vi "Average samples.vi"(6 "wait for reply (T)":bool=TRUE, 8 "error in":errorcluster, 9 "N samples":i32, 10 "Parameter":u16, 11 "Module ID":i32=-1) -> (0 "error out":errorcluster, 1 "timed out?":bool, 3 "Measurement":dbl)   [LabVIEW 2020, in "Lock-in amplifier.lvlib"]
doc: "Request to acquire multiple samples from the device. Returns the simple average of the samples.\n_____\nCreated using DQMH Event Scripter 6.1.0.128."
uses:
  Lock-in amplifier.lvlib
  Average samples Argument--cluster.ctl
  Average samples (Reply Payload)--cluster.ctl
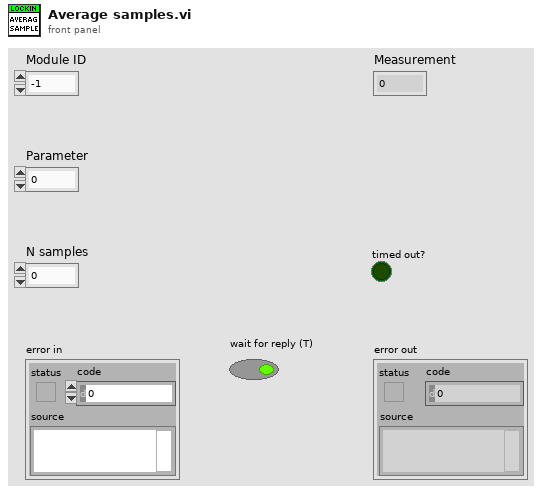
[diagram p1: front panel]
types:
  T1 = typedef "Lock-in amplifier.lvlib/Average samples Argument--cluster.ctl" = cluster{"Module ID":i32, "Parameter":u16, "N samples":i32, "Wait Notifier":refnum<notifier>, "wait for reply":bool}
  T2 = typedef "Lock-in amplifier.lvlib/Request Events--cluster.ctl" = cluster{"Stop Module":refnum<user-event>, "Show Panel":refnum<user-event>, "Hide Panel":refnum<user-event>, "Show Diagram":refnum<user-event>, "Get Module Execution Status":refnum<user-event>, "Draw Panel into Subpanel":refnum<user-event>, "Remove Panel from Subpanel":refnum<user-event>, "Connect":refnum<user-event>, "Read datapoint":refnum<user-event>, "Average samples":refnum<user-event>}
  T3 = typedef "Lock-in amplifier.lvlib/Average samples (Reply Payload)--cluster.ctl" = cluster{"Measurement":dbl, "error":errorcluster}
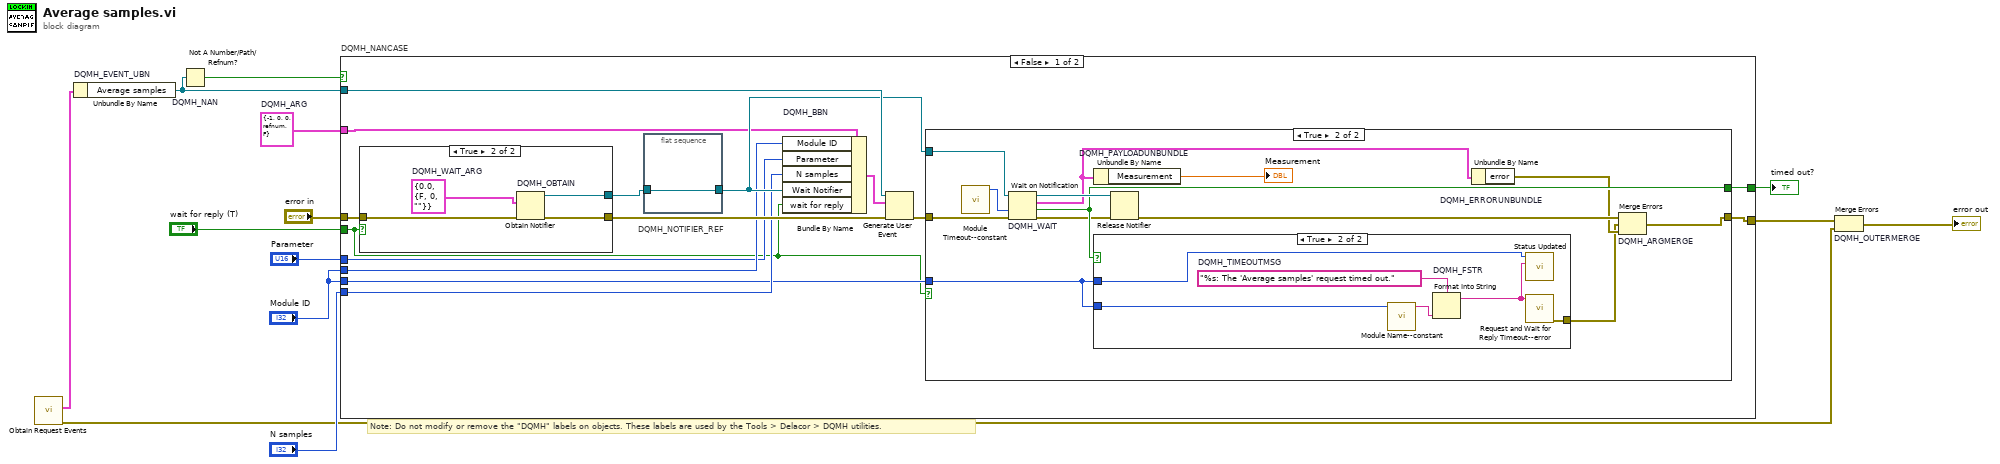
[diagram p0: block diagram]
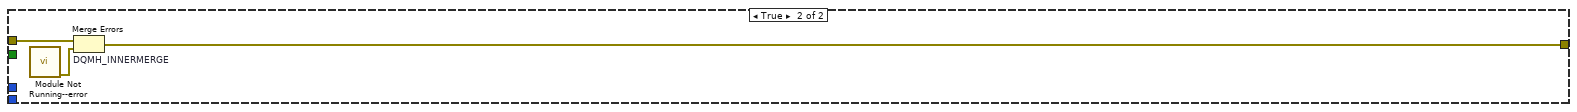
[diagram p5: hidden frame]
diagram:
  w7 = T1 {"Module ID"=-1, "Parameter"=0, "N samples"=0, "Wait Notifier"=refnum, "wait for reply"=FALSE}  # DQMH_ARG
  # "Note: Do not modify or remove the \"DQMH\" labels on objects. These labels are used by the Tools > Delacor > DQMH utilities."
  n1 = call "Obtain Request Events.vi"() -> ("error out"=w2:errorcluster, "Lock-in amplifier Request Events"=w1:T2)  [unwired: 10 in]
  n2 = Unbundle By Name "DQMH_EVENT_UBN"(w1) -> ("Average samples"=w11:refnum<user-event>)
  n3 = Not A Number/Path/Refnum? "DQMH_NAN"(number/path/refnum=w11) -> (NaN/Path/Refnum?=w10:bool)
  n4 = case "DQMH_NANCASE" shown="False" w10 {
    tunnel: "error in" -> [w28 w57]
    tunnel: w11 -> [w26 _]
    tunnel: [w23 w56] -> w8
    tunnel: [w24 _] -> w9
    tunnel: w7 -> [w19 _]
    tunnel: "Module ID" -> [w18 _]
    tunnel: "Parameter" -> [w17 _]
    tunnel: "N samples" -> [w16 _]
    tunnel: "Module ID" -> [w15 _]
    tunnel: "wait for reply (T)" -> [w14 _]
    frame False {
      n5 = case shown="True" w14 {
        tunnel: w28 -> [w50 w54]
        tunnel: [w50 w53] -> w25
        tunnel: [_ w51] -> w21
        frame False {
        }
        frame True {
          w52 = T3 {"Measurement"=0.0, "error"={"status"=FALSE, "code"=0, "source"=""}}  # DQMH_WAIT_ARG
          n6 = Obtain Notifier "DQMH_OBTAIN"(notification data type=w52, error in (no error)=w54) -> (notifier out=w51:refnum<notifier>, error out=w53:errorcluster)  [unwired: 2 in, 1 out]
        }
      }
      n7 = flat-sequence "DQMH_NOTIFIER_REF" {
        tunnel: w21 -> [w29]
        tunnel: [w29] -> w20
        frame #0 {
        }
      }
      n8 = Bundle By Name "DQMH_BBN"(cluster=w19, "Module ID"=w18, "Parameter"=w17, "N samples"=w16, "Wait Notifier"=w20, "wait for reply"=w14) -> (w22:T1)
      n9 = Generate User Event(user event=w26, event data cluster=w22, error in=w25) -> (error out=w27:errorcluster)  [unwired: 1 in, 1 out]
      n10 = case shown="True" w14 {
        tunnel: w27 -> [w30 w43]
        tunnel: w20 -> [_ w42]
        tunnel: [_ w40] -> w24
        tunnel: [w30 w39] -> w23
        tunnel: w15 -> [_ w31]
        frame False {
        }
        frame True {
          n11 = call "Module Timeout--constant.vi"() -> ("Module Timeout"=w33:i32)  [unwired: 11 in]
          n12 = Wait on Notification "DQMH_WAIT"(notifier=w42, timeout in ms (-1)=w33, error in (no error)=w43) -> (notifier out=w41:refnum<notifier>, notification=w34:T3, timed out?=w40:bool, error out=w38:errorcluster)  [unwired: 1 in]
          n13 = Unbundle By Name "DQMH_PAYLOADUNBUNDLE"(w34) -> ("Measurement"=→"Measurement":dbl)
          n14 = case shown="True" w40 {
            tunnel: [_ w47] -> w35
            tunnel: w31 -> [_ w45]
            tunnel: w31 -> [_ w44]
            frame False {
            }
            frame True {
              w49 = "%s: The 'Average samples' request timed out."  # DQMH_TIMEOUTMSG
              n15 = call "Module Name--constant.vi"("Module ID"=w44) -> ("Module Name"=w46:string)  [unwired: 10 in]
              n16 = Format Into String "DQMH_FSTR"(format string=w49, w46) -> (resulting string=w48:string)  [unwired: 2 in, 1 out]
              n17 = call "Status Updated.vi"("Status"=w48, "Module ID"=w45) -> ()  [unwired: 9 in, 1 out]
              n18 = call "Request and Wait for Reply Timeout--error.vi"("Error Message"=w48) -> ("error out"=w47:errorcluster)  [unwired: 10 in]
            }
          }
          n19 = Release Notifier(notifier=w41, error in (no error)=w38) -> (error out=w37:errorcluster)  [unwired: 1 in, 2 out]
          n20 = Unbundle By Name "DQMH_ERRORUNBUNDLE"(w34) -> ("error"=w36:errorcluster)
          n21 = Merge Errors "DQMH_ARGMERGE"(w37, w35, w36) -> (w39:errorcluster)
        }
      }
    }
    frame True {
      n22 = call "Module Not Running--error.vi"() -> ("error out"=w55:errorcluster)  [unwired: 11 in]
      n23 = Merge Errors "DQMH_INNERMERGE"(w57, w55) -> (w56:errorcluster)
    }
  }
  "timed out?" <- w9
  n24 = Merge Errors "DQMH_OUTERMERGE"(w8, w2) -> (→"error out":errorcluster)
